vi "Parse EKF_STATUS_REPORT.vi"(11 "Data":string) -> (3 "EKF Status Report":T1)   [LabVIEW 2014]
uses:
  Controls/MAVLink EKF Status Report.ctl
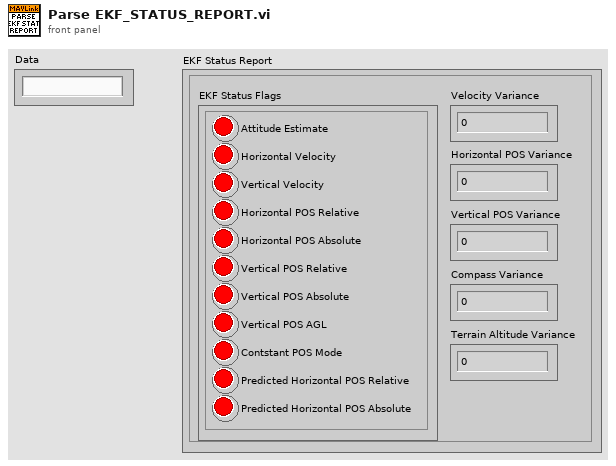
[diagram p1: front panel]
types:
  T1 = typedef "MAVLink EKF Status Report.ctl" = cluster{"EKF Status Flags":cluster{"Attitude Estimate":bool, "Horizontal Velocity":bool, "Vertical Velocity":bool, "Horizontal POS Relative":bool, "Horizontal POS Absolute":bool, "Vertical POS Relative":bool, "Vertical POS Absolute":bool, "Vertical POS AGL":bool, "Contstant POS Mode":bool, "Predicted Horizontal POS Relative":bool, "Predicted Horizontal POS Absolute":bool}, "Velocity Variance":sgl, "Horizontal POS Variance":sgl, "Vertical POS Variance":sgl, "Compass Variance":sgl, "Terrain Altitude Variance":sgl}
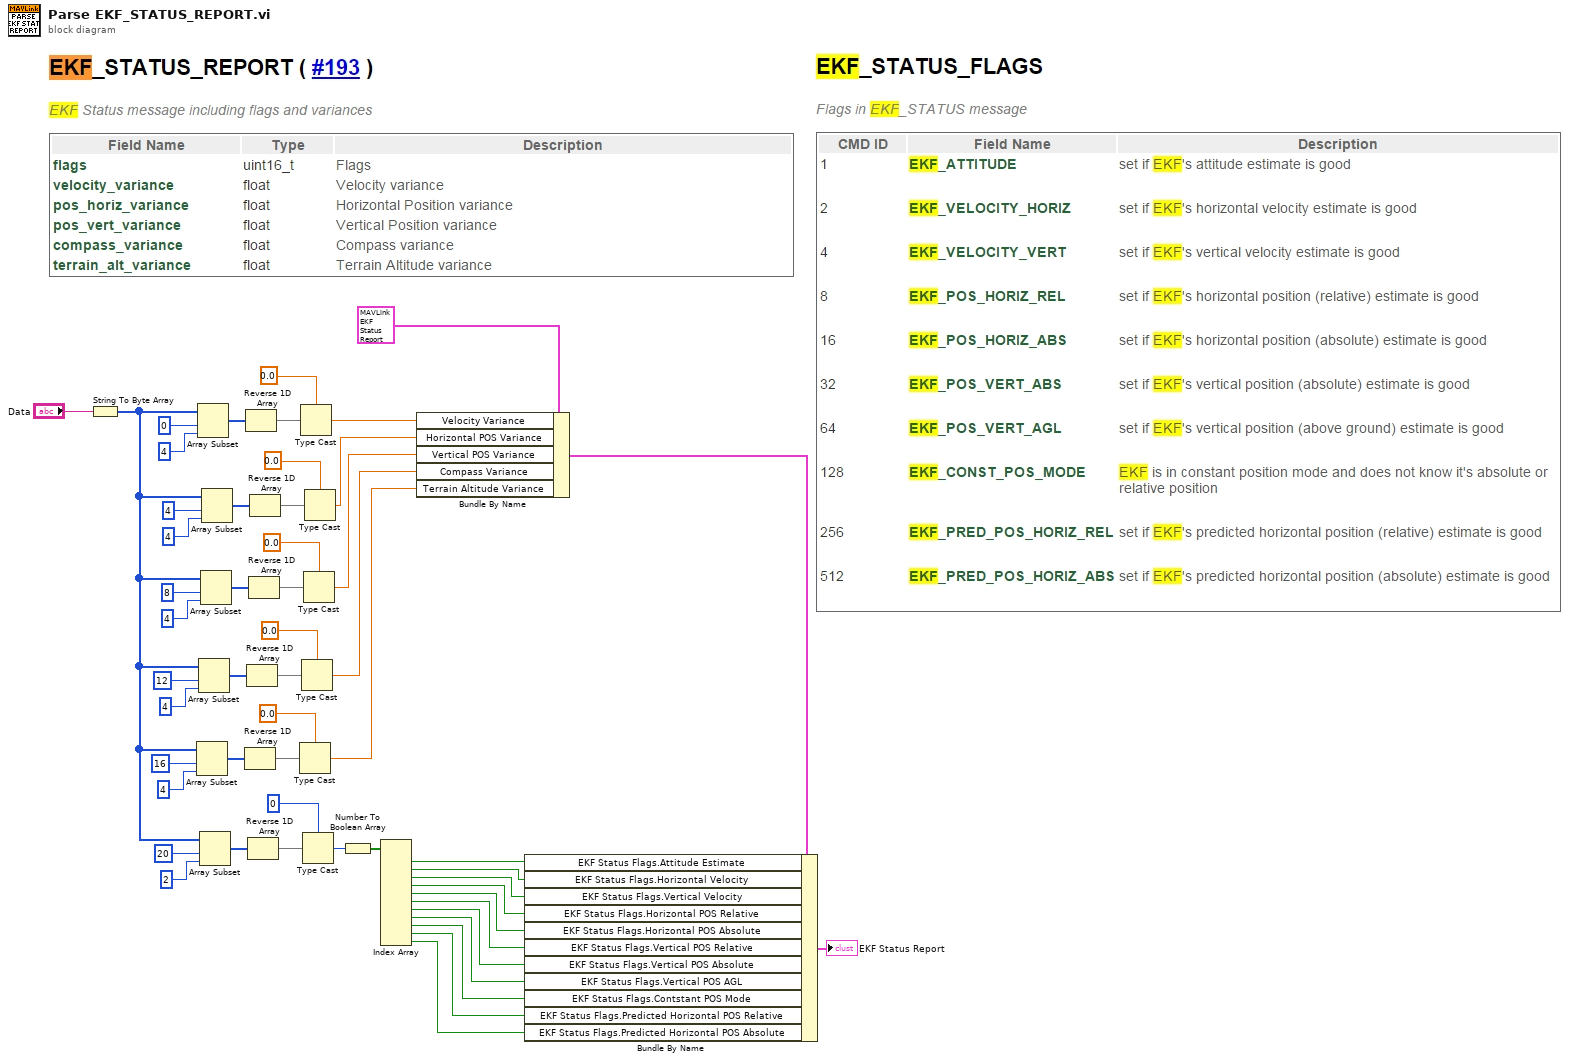
[diagram p0: block diagram]
diagram:
  n1 = String To Byte Array(string="Data") -> (unsigned byte array=w15:u8[])
  n2 = Array Subset(array=w15, index=16, length=4) -> (w25:u8[])
  n3 = Array Subset(array=w15, index=0, length=4) -> (w51:u8[])
  n4 = Array Subset(array=w15, index=12, length=4) -> (w31:u8[])
  n5 = Array Subset(array=w15, index=20, length=2) -> (w19:u8[])
  n6 = Array Subset(array=w15, index=8, length=4) -> (w37:u8[])
  n7 = Array Subset(array=w15, index=4, length=4) -> (w42:u8[])
  n8 = Reverse 1D Array(array=w25) -> (reversed array=w24:u8[])
  n9 = Reverse 1D Array(array=w51) -> (reversed array=w52:u8[])
  n10 = Reverse 1D Array(array=w31) -> (reversed array=w30:u8[])
  n11 = Reverse 1D Array(array=w19) -> (reversed array=w20:u8[])
  n12 = Reverse 1D Array(array=w37) -> (reversed array=w36:u8[])
  n13 = Reverse 1D Array(array=w42) -> (reversed array=w41:u8[])
  n14 = Type Cast(type=sgl 0.0 ("single precision float"), x=w24) -> (*(type *) &x=w22:sgl)
  n15 = Type Cast(type=sgl 0.0 ("single precision float"), x=w52) -> (*(type *) &x=w46:sgl)
  n16 = Type Cast(type=sgl 0.0 ("single precision float"), x=w30) -> (*(type *) &x=w28:sgl)
  n17 = Type Cast(type=u16 0 ("single precision float"), x=w20) -> (*(type *) &x=w14:u16)
  n18 = Type Cast(type=sgl 0.0 ("single precision float"), x=w36) -> (*(type *) &x=w34:sgl)
  n19 = Type Cast(type=sgl 0.0 ("single precision float"), x=w41) -> (*(type *) &x=w40:sgl)
  n20 = Number To Boolean Array(number=w14) -> (Boolean array=w13:bool[])
  n21 = Index Array(array=w13) -> (element #1=w12:bool, element #2=w11:bool, element #3=w10:bool, element #4=w9:bool, element #5=w8:bool, element #6=w7:bool, element #7=w6:bool, element #8=w5:bool, element #9=w4:bool, element #10=w3:bool, element #11=w2:bool)  [unwired: 11 in]
  n22 = Bundle By Name(cluster=T1 {"EKF Status Flags"={"Attitude Estimate"=FALSE, "Horizontal Velocity"=FALSE, "Vertical Velocity"=FALSE, "Horizontal POS Relative"=FALSE, "Horizontal POS Absolute"=FALSE, "Vertical POS Relative"=FALSE, "Vertical POS Absolute"=FALSE, "Vertical POS AGL"=FALSE, "Contstant POS Mode"=FALSE, "Predicted Horizontal POS Relative"=FALSE, "Predicted Horizontal POS Absolute"=FALSE}, "Velocity Variance"=0.0, "Horizontal POS Variance"=0.0, "Vertical POS Variance"=0.0, "Compass Variance"=0.0, "Terrain Altitude Variance"=0.0} ("EKF Status Report"), "Velocity Variance"=w46, "Horizontal POS Variance"=w40, "Vertical POS Variance"=w34, "Compass Variance"=w28, "Terrain Altitude Variance"=w22) -> (w21:T1)
  n23 = Bundle By Name(cluster=w21, "EKF Status Flags.Attitude Estimate"=w12, "EKF Status Flags.Horizontal Velocity"=w11, "EKF Status Flags.Vertical Velocity"=w10, "EKF Status Flags.Horizontal POS Relative"=w9, "EKF Status Flags.Horizontal POS Absolute"=w8, "EKF Status Flags.Vertical POS Relative"=w7, "EKF Status Flags.Vertical POS Absolute"=w6, "EKF Status Flags.Vertical POS AGL"=w5, "EKF Status Flags.Contstant POS Mode"=w4, "EKF Status Flags.Predicted Horizontal POS Relative"=w3, "EKF Status Flags.Predicted Horizontal POS Absolute"=w2) -> (→"EKF Status Report":T1)
